vi "testImageAnalyser2.vi"() -> ()   [LabVIEW 2011, in "run.lvlib"]
uses:
  run.lvlib
panel:
  in  "s":bool
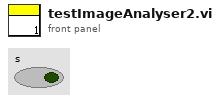
[diagram p1: front panel]
types:
  T1 = cluster{"cameraType":string, "imageName":string, "saved":string, "analysisType":string, "I16bit image data":u16[][], "path":path}
  T2 = typedef "Image Type" = u32
  T3 = typedef "IMAQ Image.ctl" = refnum<image>
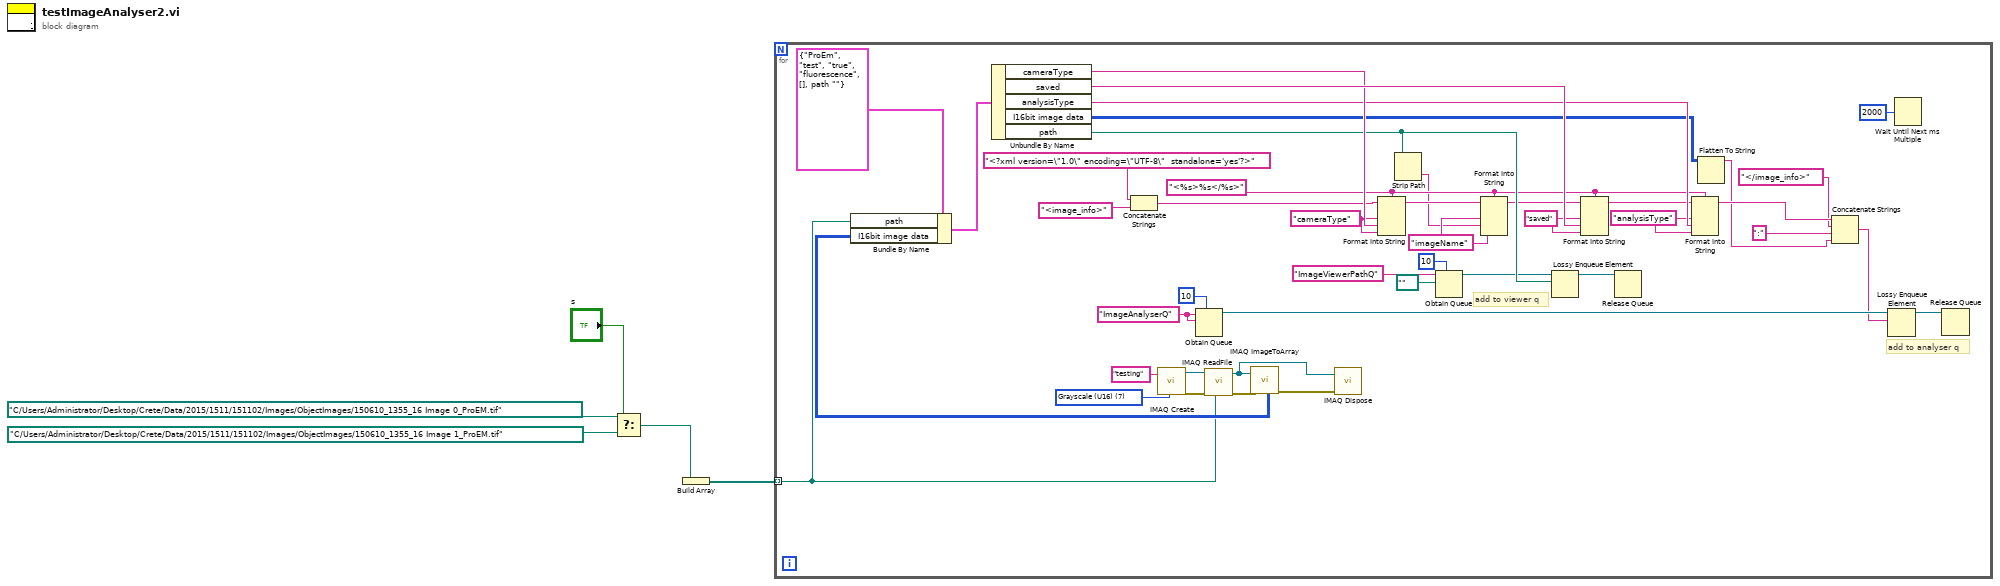
[diagram p0: block diagram]
diagram:
  n1 = Select(t=path "C:/Users/Administrator/Desktop/Crete/Data/2015/1511/151102/Images/ObjectImages/150610_1355_16 Image 0_ProEM.tif", s="s", f=path "C:/Users/Administrator/Desktop/Crete/Data/2015/1511/151102/Images/ObjectImages/150610_1355_16 Image 1_ProEM.tif") -> (s? t:f=w2:path)
  n2 = Build Array(w2) -> (w5:path[])
  n3 = for {
    tunnel: w5 -> [w8] mode=indexing
    w15 = T2 7 items=["Grayscale (U8)", "Grayscale (I16)", "Grayscale (SGL)", "Complex (CSG)", "RGB (U32)", "HSL (U32)", "RGB (U64)", "Grayscale (U16)"] ("Image Type")
    w34 = "analysisType"
    w32 = "saved"
    w28 = "imageName" ("Key")
    w27 = "cameraType"
    w39 = "ImageAnalyserQ"
    w40 = "<%s>%s</%s>"
    # "add to analyser q"
    # "add to viewer q"
    n4 = Concatenate Strings("<?xml version=\"1.0\" encoding=\"UTF-8\"  standalone='yes'?>", "<image_info>") -> (w41:string)
    n5 = call "IMAQ Create"("Image Name"="testing", "Image Type"=w15) -> ("New Image"=w14:T3, "error out"=w13:errorcluster)  [unwired: 3 in]
    n6 = Obtain Queue(max queue size (-1, unlimited)=10, name (unnamed)=w39, element data type=w39) -> (queue out=w37:refnum<queue>)  [unwired: 2 in, 2 out]
    n7 = call "IMAQ ReadFile"("File Path"=w8, "error in (no error)"=w13, "Image"=w14) -> ("error out"=w12:errorcluster, "Image Out"=w9:T3)  [unwired: 4 in, 3 out]
    n8 = call "IMAQ ImageToArray"("error in (no error)"=w12, "Image"=w9) -> ("Image Pixels (U16)"=w11:u16[][], "error out"=w10:errorcluster)  [unwired: 2 in, 3 out]
    n9 = Bundle By Name(cluster=T1 {"cameraType"="ProEm", "imageName"="test", "saved"="true", "analysisType"="fluorescence", "I16bit image data"=[], "path"=path ""} ("input cluster"), "path"=w8, "I16bit image data"=w11) -> (w17:T1)
    n10 = Unbundle By Name(w17) -> ("cameraType"=w47:string, "saved"=w48:string, "analysisType"=w46:string, "I16bit image data"=w45:u16[][], "path"=w44:path)
    n11 = call "IMAQ Dispose"("Image"=w9, "error in (no error)"=w10) -> ()  [unwired: 4 in, 1 out]
    n12 = Format Into String(format string=w40, initial string=w41, w27, w47, w27) -> (resulting string=w30:string)  [unwired: 1 in, 1 out]
    n13 = Strip Path(path=w44) -> (name=w26:string)  [unwired: 1 out]
    n14 = Obtain Queue(max queue size (-1, unlimited)=10, name (unnamed)="ImageViewerPathQ", element data type=path "") -> (queue out=w21:refnum<queue>)  [unwired: 2 in, 2 out]
    n15 = Format Into String(format string=w40, initial string=w30, w28, w26, w28) -> (resulting string=w31:string)  [unwired: 1 in, 1 out]
    n16 = Lossy Enqueue Element(queue=w21, element=w44) -> (queue out=w20:refnum<queue>)  [unwired: 1 in, 3 out]
    n17 = Format Into String(format string=w40, initial string=w31, w32, w48, w32) -> (resulting string=w35:string)  [unwired: 1 in, 1 out]
    n18 = Release Queue(queue=w20) -> ()  [unwired: 2 in, 3 out]
    n19 = Format Into String(format string=w40, initial string=w35, w34, w46, w34) -> (resulting string=w36:string)  [unwired: 1 in, 1 out]
    n20 = Flatten To String(anything=w45) -> (data string=w25:string)  [unwired: 3 in, 2 out]
    n21 = Concatenate Strings(w36, "</image_info>", ":", w25) -> (w6:string)
    n22 = Lossy Enqueue Element(queue=w37, element=w6) -> (queue out=w19:refnum<queue>)  [unwired: 1 in, 3 out]
    n23 = Wait Until Next ms Multiple(millisecond multiple=u32 2000) -> ()  [unwired: 1 out]
    n24 = Release Queue(queue=w19) -> ()  [unwired: 2 in, 3 out]
  }
